vi "ECS02_Command_Converter.vi"() -> ()   [LabVIEW 2014]
uses:
  g_CommandParam.vi
  g_ECS02_Command.vi
panel:
  out "Command to send":string
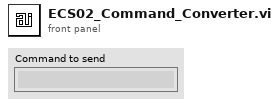
[diagram p1: front panel]
types:
  T1 = typedef "c_PlatePosEnum.ctl" = enum16{"Contact", "Seperate"}
  T2 = typedef "c_InstructionEnum.ctl" = enum16{"Move Absolute", "Increment", "Move Home", "Motion Kill", "Move Plate", "Set Stepsize", "Query Position"}
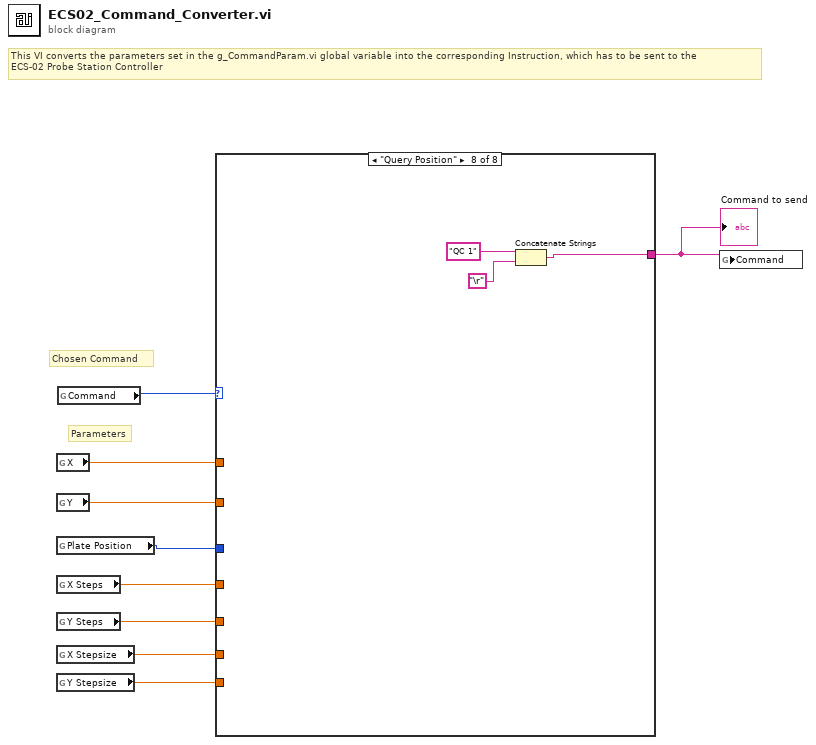
[diagram p0: block diagram]
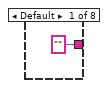
[diagram p2: hidden frame]
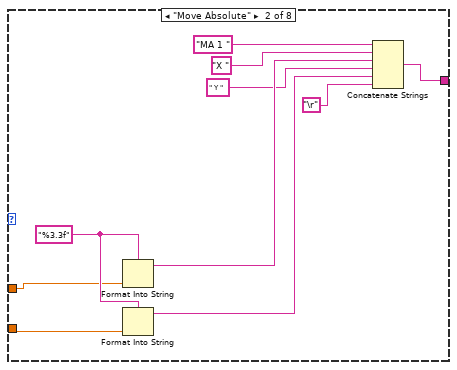
[diagram p3: hidden frame]
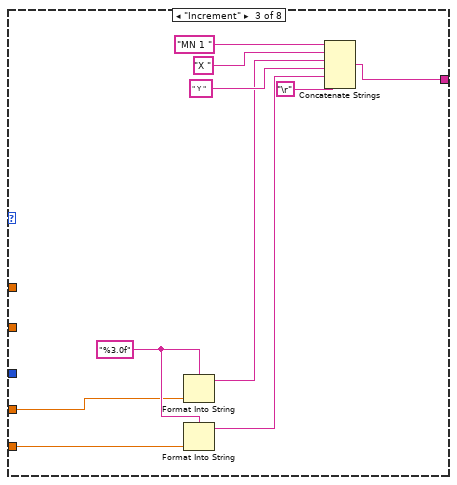
[diagram p4: hidden frame]
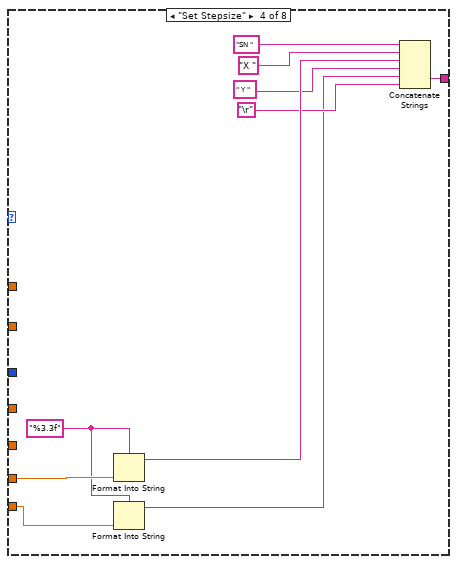
[diagram p5: hidden frame]
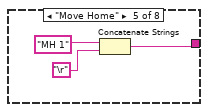
[diagram p6: hidden frame]
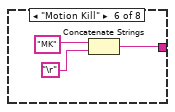
[diagram p7: hidden frame]
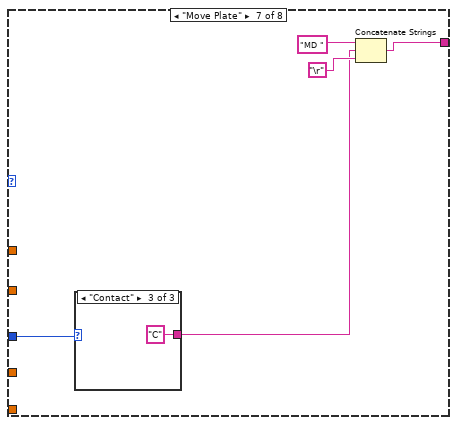
[diagram p8: hidden frame]
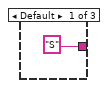
[diagram p9: hidden frame]
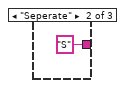
[diagram p10: hidden frame]
diagram:
  # "Parameters"
  # "Chosen Command"
  # "This VI converts the parameters set in the g_CommandParam.vi global variable into the corresponding Instruction, which has to be sent to the \nECS-02 Probe Station Controller"
  n1 = global read "g_CommandParam.vi" "X"() -> (w9:dbl)
  n2 = global read "g_CommandParam.vi" "Y"() -> (w8:dbl)
  n3 = global read "g_CommandParam.vi" "Plate Position"() -> (w1:T1)
  n4 = global read "g_CommandParam.vi" "X Steps"() -> (w7:dbl)
  n5 = global read "g_CommandParam.vi" "Y Steps"() -> (w6:dbl)
  n6 = global read "g_CommandParam.vi" "X Stepsize"() -> (w5:dbl)
  n7 = global read "g_CommandParam.vi" "Y Stepsize"() -> (w4:dbl)
  n8 = global read "g_CommandParam.vi" "Command"() -> (w2:T2)
  n9 = case shown="\"Query Position\"" w2 {
    tunnel: w9 -> [_ w16 _ _ _ _ _ _]
    tunnel: w8 -> [_ w15 _ _ _ _ _ _]
    tunnel: w7 -> [_ _ w24 _ _ _ _ _]
    tunnel: ["" w18 w26 w38 w41 w44 w48 w57] -> w3
    tunnel: w6 -> [_ _ w23 _ _ _ _ _]
    tunnel: w5 -> [_ _ _ w37 _ _ _ _]
    tunnel: w4 -> [_ _ _ w33 _ _ _ _]
    tunnel: w1 -> [_ _ _ _ _ _ w47 _]
    frame Default {
    }
    frame "Move Absolute" {
      w17 = "%3.3f" ("format string")
      n10 = Format Into String(format string=w17, w16) -> (resulting string=w14:string)  [unwired: 2 in, 1 out]
      n11 = Format Into String(format string=w17, w15) -> (resulting string=w12:string)  [unwired: 2 in, 1 out]
      n12 = Concatenate Strings("MA 1 " ("string"), "X " ("string"), w14, " Y " ("string"), w12, "\r") -> (w18:string)
    }
    frame "Increment" {
      w25 = "%3.0f" ("format string")
      n13 = Format Into String(format string=w25, w24) -> (resulting string=w21:string)  [unwired: 2 in, 1 out]
      n14 = Format Into String(format string=w25, w23) -> (resulting string=w22:string)  [unwired: 2 in, 1 out]
      n15 = Concatenate Strings("MN 1 " ("string"), "X " ("string"), w21, " Y " ("string"), w22, "\r") -> (w26:string)
    }
    frame "Set Stepsize" {
      w31 = "%3.3f" ("format string")
      n16 = Format Into String(format string=w31, w37) -> (resulting string=w36:string)  [unwired: 2 in, 1 out]
      n17 = Format Into String(format string=w31, w33) -> (resulting string=w32:string)  [unwired: 2 in, 1 out]
      n18 = Concatenate Strings("SN " ("string"), "X " ("string"), w36, " Y " ("string"), w32, "\r") -> (w38:string)
    }
    frame "Move Home" {
      n19 = Concatenate Strings("MH 1", "\r") -> (w41:string)
    }
    frame "Motion Kill" {
      n20 = Concatenate Strings("MK", "\r") -> (w44:string)
    }
    frame "Move Plate" {
      n21 = case shown="\"Contact\"" w47 {
        tunnel: ["S" "S" "C"] -> w49
        frame Default {
        }
        frame "Seperate" {
        }
        frame "Contact" {
        }
      }
      n22 = Concatenate Strings("MD ", w49, "\r") -> (w48:string)
    }
    frame "Query Position" {
      n23 = Concatenate Strings("QC 1", "\r") -> (w57:string)
    }
  }
  "Command to send" <- w3
  n24 = global write "g_ECS02_Command.vi" "Command"(w3) -> ()
